vi "Prueba_rigol.vi"(8 "error in (no error)":errorcluster, 11 "VISA IN":refnum<visa-resource-name>="FA_Rigol_DP832" caption="VISA resource name") -> (0 "error out 2":errorcluster={"status"=TRUE, "code"=-1073807360, "source"="VISA Write in Prueba_rigol.vi"}, 2 "read buffer":string)   [LabVIEW 2019]
uses:
  Rigol DP832/DP832_Control Channels.ctl
  Rigol DP832/DP832_Control Behavior.ctl
panel:
  in  "Voltage Level (0.0 V)":dbl=1.0
  in  "Current Limit (3.0 A)":dbl=0.1
  in  "Voltage Limit (6.5 V)":dbl=1.0
  out "return count 3":u32
  out "return count 2":u32
  out "return count":u32
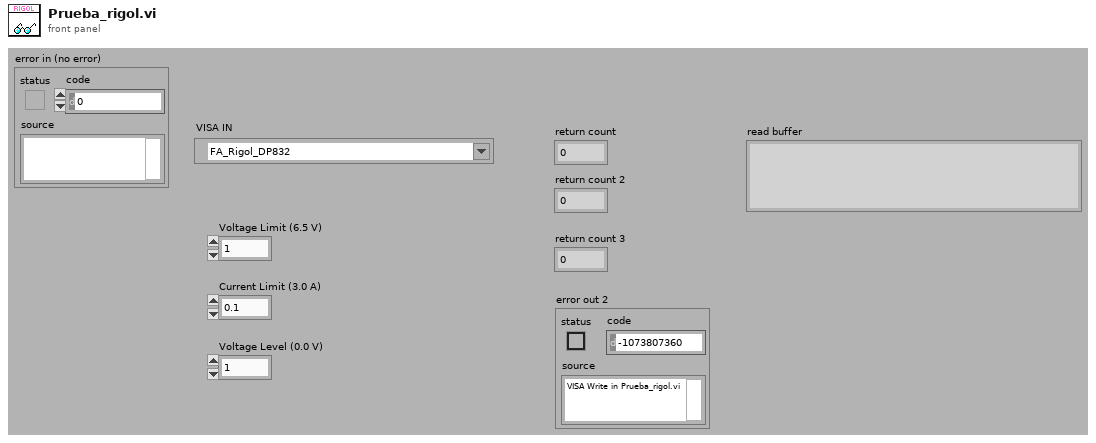
[diagram p1: front panel]
types:
  T1 = typedef "DP832_Control Behavior.ctl" = u16
  T2 = typedef "DP832_Control Channels.ctl" = i32
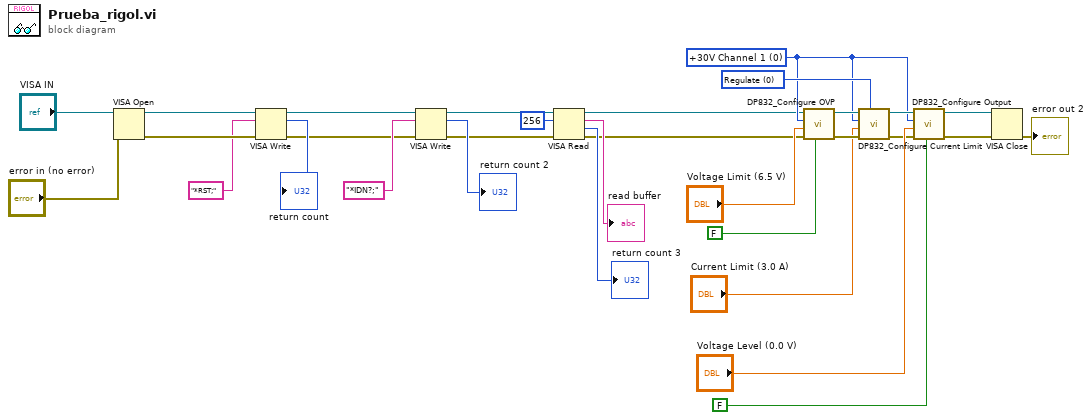
[diagram p0: block diagram]
diagram:
  w16 = T1 0 items=["Regulate", "Trip"] ("Behavior (0: Regulate)")
  w6 = T2 0 items=["+30V Channel 1", "-30V Channel 2", "+5V Channel 3"] ("Channel (0: +6V Channel)")
  n1 = VISA Open(error in (no error)="error in (no error)", VISA resource name="VISA IN") -> (VISA resource name=w29:refnum<visa-resource-name>, error out=w28:errorcluster)  [unwired: 3 in]
  n2 = VISA Write(VISA resource name=w29, write buffer="*RST;", error in (no error)=w28) -> (VISA resource name out=w23:refnum<visa-resource-name>, return count=→"return count":u32, error out=w22:errorcluster)
  n3 = VISA Write(VISA resource name=w23, write buffer="*IDN?;", error in (no error)=w22) -> (VISA resource name out=w21:refnum<visa-resource-name>, return count=→"return count 2":u32, error out=w19:errorcluster)
  n4 = VISA Read(VISA resource name=w21, byte count=u32 256, error in (no error)=w19) -> (VISA resource name out=w5:refnum<visa-resource-name>, read buffer=→"read buffer":string, return count=→"return count 3":u32, error out=w4:errorcluster)
  n5 = call "DP832_Configure OVP.vi"("Enable OVP (T: Enable)"=FALSE, "error in (no error)"=w4, "Voltage Limit"="Voltage Limit (6.5 V)", "Channel"=w6, "VISA resource name"=w5) -> ("error out"=w12:errorcluster, "VISA resource name out"=w13:refnum<visa-resource-name>)  [unwired: 5 in]
  n6 = call "DP832_Configure Current Limit.vi"("Behavior"=w16, "error in (no error)"=w12, "Current Limit"="Current Limit (3.0 A)", "Channel"=w6, "VISA resource name"=w13) -> ("error out"=w9:errorcluster, "VISA resource name out"=w8:refnum<visa-resource-name>)  [unwired: 5 in]
  n7 = call "DP832_Configure Output.vi"("Enable Output (T: Enable)"=FALSE, "error in (no error)"=w9, "Voltage Level"="Voltage Level (0.0 V)", "Channel"=w6, "VISA resource name"=w8) -> ("error out"=w2:errorcluster, "VISA resource name out"=w3:refnum<visa-resource-name>)  [unwired: 5 in]
  n8 = VISA Close(VISA resource name=w3, error in (no error)=w2) -> (error out=→"error out 2":errorcluster)
